vi "GESTISCI ESITO.vi"(0 "Esito 3 in":cluster{"Si":bool, "No":bool}, 1 "Esito 2 in":cluster{"Si":bool, "No":bool}, 2 "Esito 1 in":cluster{"Si":bool, "No":bool}, 3 "Cluster":T1, 4 "Tasto premuto":T2(array[ring]), 5 "i in":i32=1, 6 "i max":i32, 8 "Esito 4 in":cluster{"Si":bool, "No":bool}, 10 "Esito 5 in":cluster{"Si":bool, "No":bool}, 12 "Esito 6 in":cluster{"Si":bool, "No":bool}, 14 "Esito 7 in":cluster{"Si":bool, "No":bool}, 16 "Esito 8 in":cluster{"Si":bool, "No":bool}, 18 "Esito 9 in":cluster{"Si":bool, "No":bool}) -> (17 "i out":i32, 19 "Esito 9 in 2":cluster{"Si":bool, "No":bool}, 20 "Esito 1 in 2":cluster{"Si":bool, "No":bool}, 21 "Esito 2 in 2":cluster{"Si":bool, "No":bool}, 22 "Esito 3 in 2":cluster{"Si":bool, "No":bool}, 23 "Esito 4 in 2":cluster{"Si":bool, "No":bool}, 24 "Esito 5 in 2":cluster{"Si":bool, "No":bool}, 25 "Esito 6 in 2":cluster{"Si":bool, "No":bool}, 26 "Esito 7 in 2":cluster{"Si":bool, "No":bool}, 27 "Esito 8 in 2":cluster{"Si":bool, "No":bool})   [LabVIEW 2022 SP3]
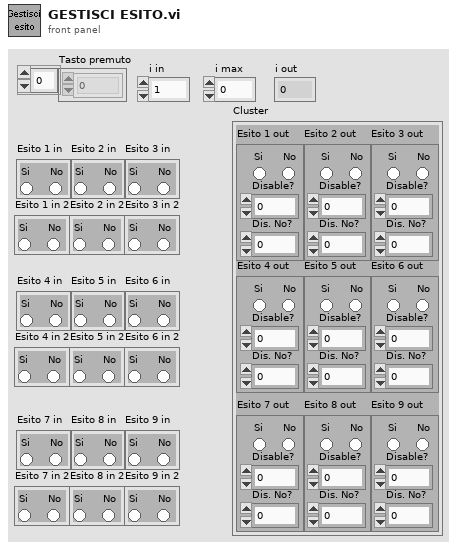
[diagram p1: front panel]
types:
  T1 = cluster{"Esito 1 out":cluster{"Disable?":i16, "Si":bool, "No":bool, "Dis. No?":i16}, "Esito 2 out":cluster{"Disable?":i16, "Si":bool, "No":bool, "Dis. No?":i16}, "Esito 3 out":cluster{"Disable?":i16, "Si":bool, "No":bool, "Dis. No?":i16}, "Esito 4 out":cluster{"Disable?":i16, "Si":bool, "No":bool, "Dis. No?":i16}, "Esito 5 out":cluster{"Disable?":i16, "Si":bool, "No":bool, "Dis. No?":i16}, "Esito 6 out":cluster{"Disable?":i16, "Si":bool, "No":bool, "Dis. No?":i16}, "Esito 7 out":cluster{"Disable?":i16, "Si":bool, "No":bool, "Dis. No?":i16}, "Esito 8 out":cluster{"Disable?":i16, "Si":bool, "No":bool, "Dis. No?":i16}, "Esito 9 out":cluster{"Disable?":i16, "Si":bool, "No":bool, "Dis. No?":i16}}
  T2 = enum16{"0", "1", "2", "3", "4", "5", "6", "7", "8", "9", "A", "B", "C", "D", "E", "F", "G", "H", "I", "J", "K", "L", "M", "N", "O", "P", "Q", "R", "S", "T", "U", "V", "W", "X", "Y", "Z", "F1", "F2", "F3", "F4", "F5", "F6", "F7", "F8", "F9", "F10", "F11", "F12", "F13", "F14", "F15", "ADD", "BACK", "BACKSLASH", "CAPITAL", "COMMA", "DECIMAL", "DELETE", "DIVIDE", "DOWN", "END", "EQUALS", "ESCAPE", "GRAVE (`)", "HOME", "INSERT", "LBRACKET", "LCONTROL", "LEFT", "L ALT", "LSHIFT", "LWIN", "MINUS", "MULTIPLY", "NEXT", "NUMLOCK", "NUMPAD_0", "NUMPAD_1", "NUMPAD_2", "NUMPAD_3", "NUMPAD_4", "NUMPAD_5", "NUMPAD_6", "NUMPAD_7", "NUMPAD_8", "NUMPAD_9", "PAUSE", "PERIOD", "PRIOR (PG UP)", "RBRACKET", "RCONTROL", "RETURN", "RIGHT", "R ALT", "RSHIFT", "RWIN", "SCROLL", "SEMICOLON", "SLASH", "SPACE", "SUBTRACT", "TAB", "UP", "ENTER (num pad)", "' (quote)"}[]
  T3 = cluster{"Disable?":i16, "Si":bool, "No":bool, "Dis. No?":i16}
  T4 = enum16{"0", "1", "2", "3", "4", "5", "6", "7", "8", "9", "A", "B", "C", "D", "E", "F", "G", "H", "I", "J", "K", "L", "M", "N", "O", "P", "Q", "R", "S", "T", "U", "V", "W", "X", "Y", "Z", "F1", "F2", "F3", "F4", "F5", "F6", "F7", "F8", "F9", "F10", "F11", "F12", "F13", "F14", "F15", "ADD", "BACK", "BACKSLASH", "CAPITAL", "COMMA", "DECIMAL", "DELETE", "DIVIDE", "DOWN", "END", "EQUALS", "ESCAPE", "GRAVE (`)", "HOME", "INSERT", "LBRACKET", "LCONTROL", "LEFT", "L ALT", "LSHIFT", "LWIN", "MINUS", "MULTIPLY", "NEXT", "NUMLOCK", "NUMPAD_0", "NUMPAD_1", "NUMPAD_2", "NUMPAD_3", "NUMPAD_4", "NUMPAD_5", "NUMPAD_6", "NUMPAD_7", "NUMPAD_8", "NUMPAD_9", "PAUSE", "PERIOD", "PRIOR (PG UP)", "RBRACKET", "RCONTROL", "RETURN", "RIGHT", "R ALT", "RSHIFT", "RWIN", "SCROLL", "SEMICOLON", "SLASH", "SPACE", "SUBTRACT", "TAB", "UP", "ENTER (num pad)", "' (quote)"}
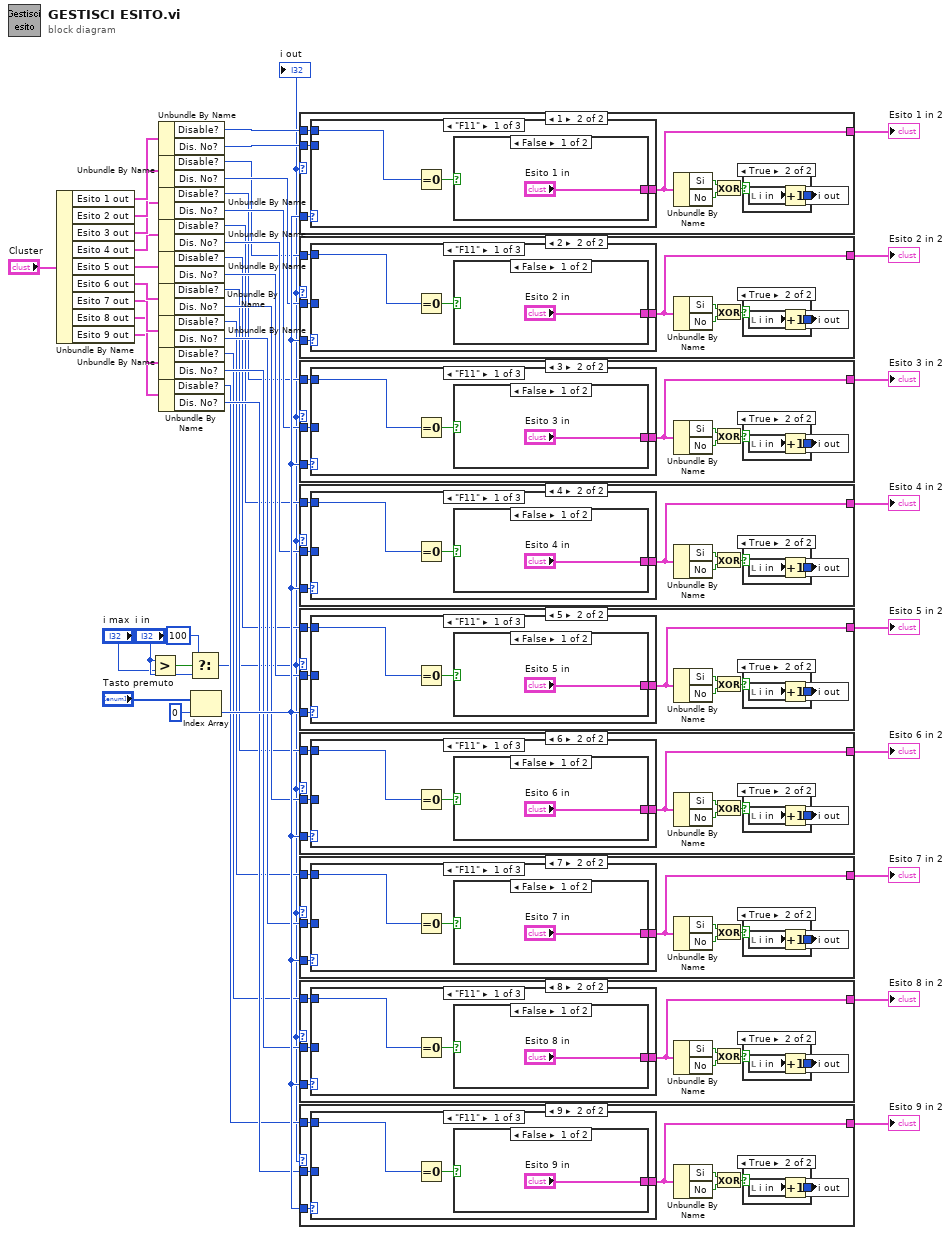
[diagram p0: block diagram]
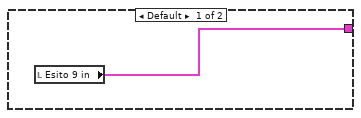
[diagram p2: hidden frame]
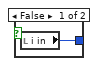
[diagram p3: hidden frame]
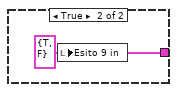
[diagram p4: hidden frame]
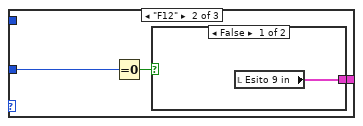
[diagram p5: hidden frame]
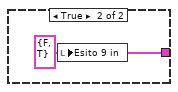
[diagram p6: hidden frame]
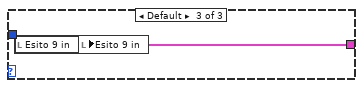
[diagram p7: hidden frame]
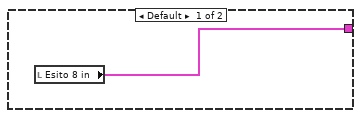
[diagram p8: hidden frame]
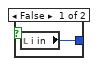
[diagram p9: hidden frame]
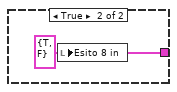
[diagram p10: hidden frame]
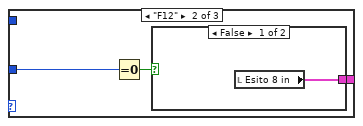
[diagram p11: hidden frame]
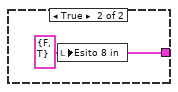
[diagram p12: hidden frame]
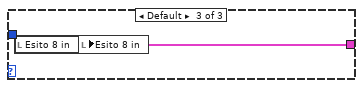
[diagram p13: hidden frame]
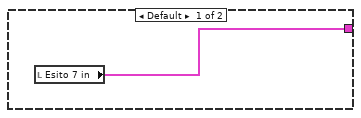
[diagram p14: hidden frame]
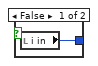
[diagram p15: hidden frame]
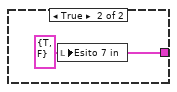
[diagram p16: hidden frame]
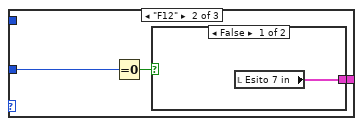
[diagram p17: hidden frame]
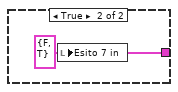
[diagram p18: hidden frame]
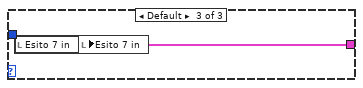
[diagram p19: hidden frame]
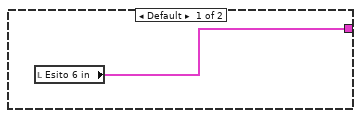
[diagram p20: hidden frame]
diagram:
  n1 = Unbundle By Name("Cluster") -> ("Esito 1 out"=w10:T3, "Esito 2 out"=w9:T3, "Esito 3 out"=w8:T3, "Esito 4 out"=w7:T3, "Esito 5 out"=w6:T3, "Esito 6 out"=w5:T3, "Esito 7 out"=w4:T3, "Esito 8 out"=w3:T3, "Esito 9 out"=w2:T3)
  n2 = Greater?(x="i in", y="i max") -> (0:w44:bool)
  n3 = Unbundle By Name(w10) -> ("Disable?"=w38:i16, "Dis. No?"=w39:i16)
  n4 = Unbundle By Name(w9) -> ("Disable?"=w29:i16, "Dis. No?"=w37:i16)
  n5 = Unbundle By Name(w8) -> ("Disable?"=w28:i16, "Dis. No?"=w36:i16)
  n6 = Unbundle By Name(w7) -> ("Disable?"=w27:i16, "Dis. No?"=w35:i16)
  n7 = Unbundle By Name(w6) -> ("Disable?"=w26:i16, "Dis. No?"=w34:i16)
  n8 = Unbundle By Name(w5) -> ("Disable?"=w25:i16, "Dis. No?"=w33:i16)
  n9 = Unbundle By Name(w4) -> ("Disable?"=w24:i16, "Dis. No?"=w32:i16)
  n10 = Unbundle By Name(w3) -> ("Disable?"=w23:i16, "Dis. No?"=w31:i16)
  n11 = Unbundle By Name(w2) -> ("Disable?"=w22:i16, "Dis. No?"=w30:i16)
  n12 = Select(t=100, s=w44, f="i in") -> (s? t:f=w1:i32)
  "i out" <- w1
  n13 = Index Array(array="Tasto premuto", index=0) -> (element=w40:T4)
  n14 = case shown="1" w1 {
    tunnel: w40 -> [_ w50]
    tunnel: [w46 w49] -> w20
    tunnel: w39 -> [_ w48]
    tunnel: w38 -> [_ w47]
    frame Default {
      n15 = local read "Esito 1 in"() -> (w46:cluster{"Si":bool, "No":bool})
    }
    frame 1 {
      n16 = case shown="\"F11\"" w50 {
        tunnel: [w60 w65 w68] -> w49
        tunnel: w48 -> [_ w63 _]
        tunnel: w47 -> [w58 _ _]
        frame "F11" {
          n17 = Equal To 0?(x=w58) -> (x = 0?=w59:bool)
          n18 = case shown="False" w59 {
            tunnel: ["Esito 1 in" w62] -> w60
            frame False {
            }
            frame True {
              w62 = cluster{"Si":bool, "No":bool} {"Si"=TRUE, "No"=FALSE} ("Si/No 1")
              n19 = local write "Esito 1 in"(w62) -> ()
            }
          }
        }
        frame "F12" {
          n20 = Equal To 0?(x=w63) -> (x = 0?=w64:bool)
          n21 = case shown="False" w64 {
            tunnel: [w66 w67] -> w65
            frame False {
              n22 = local read "Esito 1 in"() -> (w66:cluster{"Si":bool, "No":bool})
            }
            frame True {
              w67 = cluster{"Si":bool, "No":bool} {"Si"=FALSE, "No"=TRUE} ("Si/No 1")
              n23 = local write "Esito 1 in"(w67) -> ()
            }
          }
        }
        frame Default {
          n24 = local read "Esito 1 in"() -> (w68:cluster{"Si":bool, "No":bool})
          n25 = local write "Esito 1 in"(w68) -> ()
        }
      }
      n26 = Unbundle By Name(w49) -> ("Si"=w53:bool, "No"=w54:bool)
      n27 = Exclusive Or(1:w54, 2:w53) -> (0:w52:bool)
      n28 = case shown="True" w52 {
        tunnel: [w55 w57] -> w51
        frame False {
          n29 = local read "i in"() -> (w55:i32)
        }
        frame True {
          n30 = local read "i in"() -> (w56:i32)
          n31 = Increment(x=w56) -> (x+1=w57:i32)
        }
      }
      n32 = local write "i out"(w51) -> ()
    }
  }
  "Esito 1 in 2" <- w20
  n33 = case shown="2" w1 {
    tunnel: w40 -> [_ w73]
    tunnel: [w69 w72] -> w19
    tunnel: w37 -> [_ w71]
    tunnel: w29 -> [_ w70]
    frame Default {
      n34 = local read "Esito 2 in"() -> (w69:cluster{"Si":bool, "No":bool})
    }
    frame 2 {
      n35 = case shown="\"F11\"" w73 {
        tunnel: [w83 w88 w91] -> w72
        tunnel: w71 -> [_ w86 _]
        tunnel: w70 -> [w81 _ _]
        frame "F11" {
          n36 = Equal To 0?(x=w81) -> (x = 0?=w82:bool)
          n37 = case shown="False" w82 {
            tunnel: ["Esito 2 in" w85] -> w83
            frame False {
            }
            frame True {
              w85 = cluster{"Si":bool, "No":bool} {"Si"=TRUE, "No"=FALSE} ("Si/No 1")
              n38 = local write "Esito 2 in"(w85) -> ()
            }
          }
        }
        frame "F12" {
          n39 = Equal To 0?(x=w86) -> (x = 0?=w87:bool)
          n40 = case shown="False" w87 {
            tunnel: [w89 w90] -> w88
            frame False {
              n41 = local read "Esito 2 in"() -> (w89:cluster{"Si":bool, "No":bool})
            }
            frame True {
              w90 = cluster{"Si":bool, "No":bool} {"Si"=FALSE, "No"=TRUE} ("Si/No 1")
              n42 = local write "Esito 2 in"(w90) -> ()
            }
          }
        }
        frame Default {
          n43 = local read "Esito 2 in"() -> (w91:cluster{"Si":bool, "No":bool})
          n44 = local write "Esito 2 in"(w91) -> ()
        }
      }
      n45 = Unbundle By Name(w72) -> ("Si"=w76:bool, "No"=w77:bool)
      n46 = Exclusive Or(1:w77, 2:w76) -> (0:w75:bool)
      n47 = case shown="True" w75 {
        tunnel: [w78 w80] -> w74
        frame False {
          n48 = local read "i in"() -> (w78:i32)
        }
        frame True {
          n49 = local read "i in"() -> (w79:i32)
          n50 = Increment(x=w79) -> (x+1=w80:i32)
        }
      }
      n51 = local write "i out"(w74) -> ()
    }
  }
  "Esito 2 in 2" <- w19
  n52 = case shown="3" w1 {
    tunnel: w40 -> [_ w96]
    tunnel: [w92 w95] -> w18
    tunnel: w36 -> [_ w94]
    tunnel: w28 -> [_ w93]
    frame Default {
      n53 = local read "Esito 3 in"() -> (w92:cluster{"Si":bool, "No":bool})
    }
    frame 3 {
      n54 = case shown="\"F11\"" w96 {
        tunnel: [w106 w111 w114] -> w95
        tunnel: w94 -> [_ w109 _]
        tunnel: w93 -> [w104 _ _]
        frame "F11" {
          n55 = Equal To 0?(x=w104) -> (x = 0?=w105:bool)
          n56 = case shown="False" w105 {
            tunnel: ["Esito 3 in" w108] -> w106
            frame False {
            }
            frame True {
              w108 = cluster{"Si":bool, "No":bool} {"Si"=TRUE, "No"=FALSE} ("Si/No 1")
              n57 = local write "Esito 3 in"(w108) -> ()
            }
          }
        }
        frame "F12" {
          n58 = Equal To 0?(x=w109) -> (x = 0?=w110:bool)
          n59 = case shown="False" w110 {
            tunnel: [w112 w113] -> w111
            frame False {
              n60 = local read "Esito 3 in"() -> (w112:cluster{"Si":bool, "No":bool})
            }
            frame True {
              w113 = cluster{"Si":bool, "No":bool} {"Si"=FALSE, "No"=TRUE} ("Si/No 1")
              n61 = local write "Esito 3 in"(w113) -> ()
            }
          }
        }
        frame Default {
          n62 = local read "Esito 3 in"() -> (w114:cluster{"Si":bool, "No":bool})
          n63 = local write "Esito 3 in"(w114) -> ()
        }
      }
      n64 = Unbundle By Name(w95) -> ("Si"=w99:bool, "No"=w100:bool)
      n65 = Exclusive Or(1:w100, 2:w99) -> (0:w98:bool)
      n66 = case shown="True" w98 {
        tunnel: [w101 w103] -> w97
        frame False {
          n67 = local read "i in"() -> (w101:i32)
        }
        frame True {
          n68 = local read "i in"() -> (w102:i32)
          n69 = Increment(x=w102) -> (x+1=w103:i32)
        }
      }
      n70 = local write "i out"(w97) -> ()
    }
  }
  "Esito 3 in 2" <- w18
  n71 = case shown="4" w1 {
    tunnel: w40 -> [_ w119]
    tunnel: [w115 w118] -> w17
    tunnel: w35 -> [_ w117]
    tunnel: w27 -> [_ w116]
    frame Default {
      n72 = local read "Esito 4 in"() -> (w115:cluster{"Si":bool, "No":bool})
    }
    frame 4 {
      n73 = case shown="\"F11\"" w119 {
        tunnel: [w129 w134 w137] -> w118
        tunnel: w117 -> [_ w132 _]
        tunnel: w116 -> [w127 _ _]
        frame "F11" {
          n74 = Equal To 0?(x=w127) -> (x = 0?=w128:bool)
          n75 = case shown="False" w128 {
            tunnel: ["Esito 4 in" w131] -> w129
            frame False {
            }
            frame True {
              w131 = cluster{"Si":bool, "No":bool} {"Si"=TRUE, "No"=FALSE} ("Si/No 1")
              n76 = local write "Esito 4 in"(w131) -> ()
            }
          }
        }
        frame "F12" {
          n77 = Equal To 0?(x=w132) -> (x = 0?=w133:bool)
          n78 = case shown="False" w133 {
            tunnel: [w135 w136] -> w134
            frame False {
              n79 = local read "Esito 4 in"() -> (w135:cluster{"Si":bool, "No":bool})
            }
            frame True {
              w136 = cluster{"Si":bool, "No":bool} {"Si"=FALSE, "No"=TRUE} ("Si/No 1")
              n80 = local write "Esito 4 in"(w136) -> ()
            }
          }
        }
        frame Default {
          n81 = local read "Esito 4 in"() -> (w137:cluster{"Si":bool, "No":bool})
          n82 = local write "Esito 4 in"(w137) -> ()
        }
      }
      n83 = Unbundle By Name(w118) -> ("Si"=w122:bool, "No"=w123:bool)
      n84 = Exclusive Or(1:w123, 2:w122) -> (0:w121:bool)
      n85 = case shown="True" w121 {
        tunnel: [w124 w126] -> w120
        frame False {
          n86 = local read "i in"() -> (w124:i32)
        }
        frame True {
          n87 = local read "i in"() -> (w125:i32)
          n88 = Increment(x=w125) -> (x+1=w126:i32)
        }
      }
      n89 = local write "i out"(w120) -> ()
    }
  }
  "Esito 4 in 2" <- w17
  n90 = case shown="5" w1 {
    tunnel: w40 -> [_ w142]
    tunnel: [w138 w141] -> w16
    tunnel: w34 -> [_ w140]
    tunnel: w26 -> [_ w139]
    frame Default {
      n91 = local read "Esito 5 in"() -> (w138:cluster{"Si":bool, "No":bool})
    }
    frame 5 {
      n92 = case shown="\"F11\"" w142 {
        tunnel: [w152 w157 w160] -> w141
        tunnel: w140 -> [_ w155 _]
        tunnel: w139 -> [w150 _ _]
        frame "F11" {
          n93 = Equal To 0?(x=w150) -> (x = 0?=w151:bool)
          n94 = case shown="False" w151 {
            tunnel: ["Esito 5 in" w154] -> w152
            frame False {
            }
            frame True {
              w154 = cluster{"Si":bool, "No":bool} {"Si"=TRUE, "No"=FALSE} ("Si/No 1")
              n95 = local write "Esito 5 in"(w154) -> ()
            }
          }
        }
        frame "F12" {
          n96 = Equal To 0?(x=w155) -> (x = 0?=w156:bool)
          n97 = case shown="False" w156 {
            tunnel: [w158 w159] -> w157
            frame False {
              n98 = local read "Esito 5 in"() -> (w158:cluster{"Si":bool, "No":bool})
            }
            frame True {
              w159 = cluster{"Si":bool, "No":bool} {"Si"=FALSE, "No"=TRUE} ("Si/No 1")
              n99 = local write "Esito 5 in"(w159) -> ()
            }
          }
        }
        frame Default {
          n100 = local read "Esito 5 in"() -> (w160:cluster{"Si":bool, "No":bool})
          n101 = local write "Esito 5 in"(w160) -> ()
        }
      }
      n102 = Unbundle By Name(w141) -> ("Si"=w145:bool, "No"=w146:bool)
      n103 = Exclusive Or(1:w146, 2:w145) -> (0:w144:bool)
      n104 = case shown="True" w144 {
        tunnel: [w147 w149] -> w143
        frame False {
          n105 = local read "i in"() -> (w147:i32)
        }
        frame True {
          n106 = local read "i in"() -> (w148:i32)
          n107 = Increment(x=w148) -> (x+1=w149:i32)
        }
      }
      n108 = local write "i out"(w143) -> ()
    }
  }
  "Esito 5 in 2" <- w16
  n109 = case shown="6" w1 {
    tunnel: w40 -> [_ w165]
    tunnel: [w161 w164] -> w15
    tunnel: w33 -> [_ w163]
    tunnel: w25 -> [_ w162]
    frame Default {
      n110 = local read "Esito 6 in"() -> (w161:cluster{"Si":bool, "No":bool})
    }
    frame 6 {
      n111 = case shown="\"F11\"" w165 {
        tunnel: [w175 w180 w183] -> w164
        tunnel: w163 -> [_ w178 _]
        tunnel: w162 -> [w173 _ _]
        frame "F11" {
          n112 = Equal To 0?(x=w173) -> (x = 0?=w174:bool)
          n113 = case shown="False" w174 {
            tunnel: ["Esito 6 in" w177] -> w175
            frame False {
            }
            frame True {
              w177 = cluster{"Si":bool, "No":bool} {"Si"=TRUE, "No"=FALSE} ("Si/No 1")
              n114 = local write "Esito 6 in"(w177) -> ()
            }
          }
        }
        frame "F12" {
          n115 = Equal To 0?(x=w178) -> (x = 0?=w179:bool)
          n116 = case shown="False" w179 {
            tunnel: [w181 w182] -> w180
            frame False {
              n117 = local read "Esito 6 in"() -> (w181:cluster{"Si":bool, "No":bool})
            }
            frame True {
              w182 = cluster{"Si":bool, "No":bool} {"Si"=FALSE, "No"=TRUE} ("Si/No 1")
              n118 = local write "Esito 6 in"(w182) -> ()
            }
          }
        }
        frame Default {
          n119 = local read "Esito 6 in"() -> (w183:cluster{"Si":bool, "No":bool})
          n120 = local write "Esito 6 in"(w183) -> ()
        }
      }
      n121 = Unbundle By Name(w164) -> ("Si"=w168:bool, "No"=w169:bool)
      n122 = Exclusive Or(1:w169, 2:w168) -> (0:w167:bool)
      n123 = case shown="True" w167 {
        tunnel: [w170 w172] -> w166
        frame False {
          n124 = local read "i in"() -> (w170:i32)
        }
        frame True {
          n125 = local read "i in"() -> (w171:i32)
          n126 = Increment(x=w171) -> (x+1=w172:i32)
        }
      }
      n127 = local write "i out"(w166) -> ()
    }
  }
  "Esito 6 in 2" <- w15
  n128 = case shown="7" w1 {
    tunnel: w40 -> [_ w188]
    tunnel: [w184 w187] -> w14
    tunnel: w32 -> [_ w186]
    tunnel: w24 -> [_ w185]
    frame Default {
      n129 = local read "Esito 7 in"() -> (w184:cluster{"Si":bool, "No":bool})
    }
    frame 7 {
      n130 = case shown="\"F11\"" w188 {
        tunnel: [w198 w203 w206] -> w187
        tunnel: w186 -> [_ w201 _]
        tunnel: w185 -> [w196 _ _]
        frame "F11" {
          n131 = Equal To 0?(x=w196) -> (x = 0?=w197:bool)
          n132 = case shown="False" w197 {
            tunnel: ["Esito 7 in" w200] -> w198
            frame False {
            }
            frame True {
              w200 = cluster{"Si":bool, "No":bool} {"Si"=TRUE, "No"=FALSE} ("Si/No 1")
              n133 = local write "Esito 7 in"(w200) -> ()
            }
          }
        }
        frame "F12" {
          n134 = Equal To 0?(x=w201) -> (x = 0?=w202:bool)
          n135 = case shown="False" w202 {
            tunnel: [w204 w205] -> w203
            frame False {
              n136 = local read "Esito 7 in"() -> (w204:cluster{"Si":bool, "No":bool})
            }
            frame True {
              w205 = cluster{"Si":bool, "No":bool} {"Si"=FALSE, "No"=TRUE} ("Si/No 1")
              n137 = local write "Esito 7 in"(w205) -> ()
            }
          }
        }
        frame Default {
          n138 = local read "Esito 7 in"() -> (w206:cluster{"Si":bool, "No":bool})
          n139 = local write "Esito 7 in"(w206) -> ()
        }
      }
      n140 = Unbundle By Name(w187) -> ("Si"=w191:bool, "No"=w192:bool)
      n141 = Exclusive Or(1:w192, 2:w191) -> (0:w190:bool)
      n142 = case shown="True" w190 {
        tunnel: [w193 w195] -> w189
        frame False {
          n143 = local read "i in"() -> (w193:i32)
        }
        frame True {
          n144 = local read "i in"() -> (w194:i32)
          n145 = Increment(x=w194) -> (x+1=w195:i32)
        }
      }
      n146 = local write "i out"(w189) -> ()
    }
  }
  "Esito 7 in 2" <- w14
  n147 = case shown="8" w1 {
    tunnel: w40 -> [_ w211]
    tunnel: [w207 w210] -> w13
    tunnel: w31 -> [_ w209]
    tunnel: w23 -> [_ w208]
    frame Default {
      n148 = local read "Esito 8 in"() -> (w207:cluster{"Si":bool, "No":bool})
    }
    frame 8 {
      n149 = case shown="\"F11\"" w211 {
        tunnel: [w221 w226 w229] -> w210
        tunnel: w209 -> [_ w224 _]
        tunnel: w208 -> [w219 _ _]
        frame "F11" {
          n150 = Equal To 0?(x=w219) -> (x = 0?=w220:bool)
          n151 = case shown="False" w220 {
            tunnel: ["Esito 8 in" w223] -> w221
            frame False {
            }
            frame True {
              w223 = cluster{"Si":bool, "No":bool} {"Si"=TRUE, "No"=FALSE} ("Si/No 1")
              n152 = local write "Esito 8 in"(w223) -> ()
            }
          }
        }
        frame "F12" {
          n153 = Equal To 0?(x=w224) -> (x = 0?=w225:bool)
          n154 = case shown="False" w225 {
            tunnel: [w227 w228] -> w226
            frame False {
              n155 = local read "Esito 8 in"() -> (w227:cluster{"Si":bool, "No":bool})
            }
            frame True {
              w228 = cluster{"Si":bool, "No":bool} {"Si"=FALSE, "No"=TRUE} ("Si/No 1")
              n156 = local write "Esito 8 in"(w228) -> ()
            }
          }
        }
        frame Default {
          n157 = local read "Esito 8 in"() -> (w229:cluster{"Si":bool, "No":bool})
          n158 = local write "Esito 8 in"(w229) -> ()
        }
      }
      n159 = Unbundle By Name(w210) -> ("Si"=w214:bool, "No"=w215:bool)
      n160 = Exclusive Or(1:w215, 2:w214) -> (0:w213:bool)
      n161 = case shown="True" w213 {
        tunnel: [w216 w218] -> w212
        frame False {
          n162 = local read "i in"() -> (w216:i32)
        }
        frame True {
          n163 = local read "i in"() -> (w217:i32)
          n164 = Increment(x=w217) -> (x+1=w218:i32)
        }
      }
      n165 = local write "i out"(w212) -> ()
    }
  }
  "Esito 8 in 2" <- w13
  n166 = case shown="9" w1 {
    tunnel: w40 -> [_ w234]
    tunnel: [w230 w233] -> w12
    tunnel: w30 -> [_ w232]
    tunnel: w22 -> [_ w231]
    frame Default {
      n167 = local read "Esito 9 in"() -> (w230:cluster{"Si":bool, "No":bool})
    }
    frame 9 {
      n168 = case shown="\"F11\"" w234 {
        tunnel: [w244 w249 w252] -> w233
        tunnel: w232 -> [_ w247 _]
        tunnel: w231 -> [w242 _ _]
        frame "F11" {
          n169 = Equal To 0?(x=w242) -> (x = 0?=w243:bool)
          n170 = case shown="False" w243 {
            tunnel: ["Esito 9 in" w246] -> w244
            frame False {
            }
            frame True {
              w246 = cluster{"Si":bool, "No":bool} {"Si"=TRUE, "No"=FALSE} ("Si/No 1")
              n171 = local write "Esito 9 in"(w246) -> ()
            }
          }
        }
        frame "F12" {
          n172 = Equal To 0?(x=w247) -> (x = 0?=w248:bool)
          n173 = case shown="False" w248 {
            tunnel: [w250 w251] -> w249
            frame False {
              n174 = local read "Esito 9 in"() -> (w250:cluster{"Si":bool, "No":bool})
            }
            frame True {
              w251 = cluster{"Si":bool, "No":bool} {"Si"=FALSE, "No"=TRUE} ("Si/No 1")
              n175 = local write "Esito 9 in"(w251) -> ()
            }
          }
        }
        frame Default {
          n176 = local read "Esito 9 in"() -> (w252:cluster{"Si":bool, "No":bool})
          n177 = local write "Esito 9 in"(w252) -> ()
        }
      }
      n178 = Unbundle By Name(w233) -> ("Si"=w237:bool, "No"=w238:bool)
      n179 = Exclusive Or(1:w238, 2:w237) -> (0:w236:bool)
      n180 = case shown="True" w236 {
        tunnel: [w239 w241] -> w235
        frame False {
          n181 = local read "i in"() -> (w239:i32)
        }
        frame True {
          n182 = local read "i in"() -> (w240:i32)
          n183 = Increment(x=w240) -> (x+1=w241:i32)
        }
      }
      n184 = local write "i out"(w235) -> ()
    }
  }
  "Esito 9 in 2" <- w12
